vi "get_alignment_mode.vi"(8 "error in (no error)":errorcluster, 11 "LightSourceAN191011Chameleon in":refnum<class "LightSourceAN191011Chameleon.lvclass">) -> (0 "error out":errorcluster, 2 "alignment mode?":bool, 3 "LightSourceAN191011Chameleon out":refnum<class "LightSourceAN191011Chameleon.lvclass">)   [LabVIEW 2010, in "LightSourceAN191011Chameleon.lvclass"]
uses:
  LightSourceAN191011Chameleon.lvclass
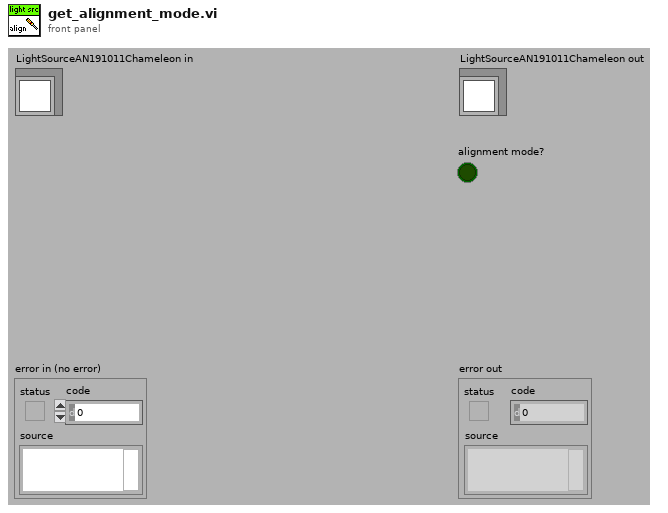
[diagram p1: front panel]
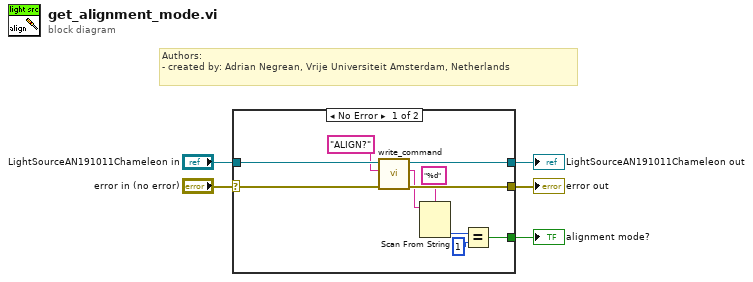
[diagram p0: block diagram]
diagram:
  # "Authors: \n- created by: Adrian Negrean, Vrije Universiteit Amsterdam, Netherlands"
  n1 = case shown="No Error" "error in (no error)" {
    selector: "error in (no error)" -> [w13 w17]
    tunnel: [w12 w17] -> w4
    tunnel: [w14 w16] -> w2
    tunnel: "LightSourceAN191011Chameleon in" -> [w15 w16]
    tunnel: [w6 _] -> w1
    frame No Error {
      n2 = call-dynamic "write_command.vi"("error in (no error)"=w13, "string to write"="ALIGN?" ("string"), "LightSourceAN191011Chameleon in"=w15) -> ("error out"=w12:errorcluster, "read string"=w10:string, "LightSourceAN191011Chameleon out"=w14:refnum<class "LightSourceAN191011Chameleon.lvclass">)  [unwired: 6 in]
      n3 = Scan From String(format string="%d", input string=w10) -> (output 1=w8:i32)  [unwired: 3 in, 3 out]
      n4 = Equal?(x=w8, y=1) -> (x = y?=w6:bool)
    }
    frame Error {
    }
  }
  "error out" <- w4
  "LightSourceAN191011Chameleon out" <- w2
  "alignment mode?" <- w1
